vi "BallShear_PackageAnalysis.vi"(4 "Real Coordinates":path=path "C:/Users/Nicole/Documents/GitHub/Ball_Shear/0_BallShear/data/rcoord.csv", 5 "Virtual Coordinates":path=path "C:/Users/Nicole/Documents/GitHub/Ball_Shear/0_BallShear/data/vcoord.csv", 6 "Coord Conversion Script":path=path "C:/Users/Nicole/Documents/GitHub/Ball_Shear/0_BallShear/scripts/coordinate_conversion.py", 7 "Package Analysis Script":path=path "C:/Users/Nicole/Documents/GitHub/Ball_Shear/0_BallShear/scripts/pixel_location.py", 9 "Analyzed Package Path":path=path "C:/Users/Nicole/Documents/GitHub/Ball_Shear/0_BallShear/img/packageAnalyzed.png", 10 "Original Package Path":path=path "C:/Users/Nicole/Documents/GitHub/Ball_Shear/0_BallShear/img/package.png", 11 "Analyze":bool) -> (0 "Displayed Path":path, 1 "IDs":string[](array[string]), 2 "Coordinates":dbl[][](array[numeric]), 3 "Success":bool)   [LabVIEW 2013]
uses:
  <vilib>/Utility/file.llb/Read From Spreadsheet File (DBL).vi
panel:
  out "all rows":dbl[][](array[numeric]) format="%0.3f"
  out "return code 2":i32
  out "standard error 2":string
  out "standard output 2":string
  out "Command 2":string
  out "Command":string
  out "return code":i32
  out "standard error":string
  out "standard output":string
  # "Ball Detection"
  # "Coordinate Conversion"
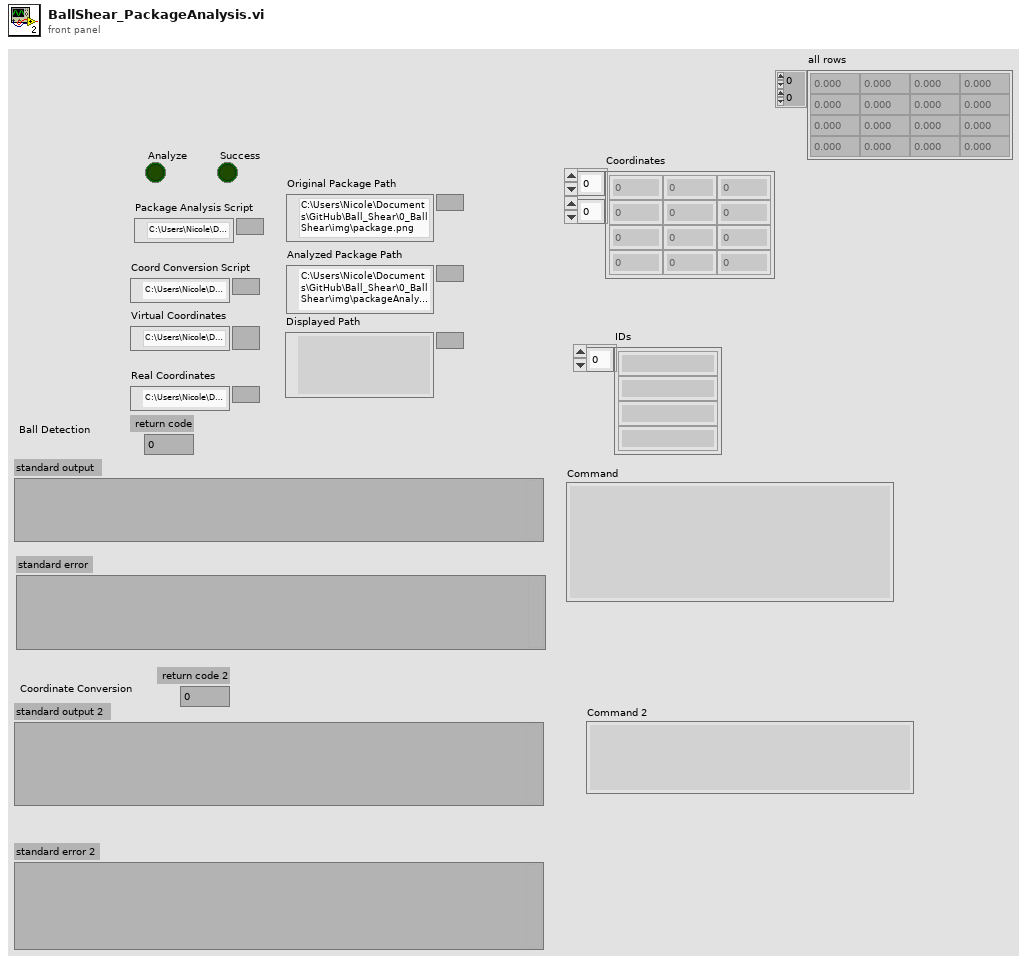
[diagram p1: front panel]
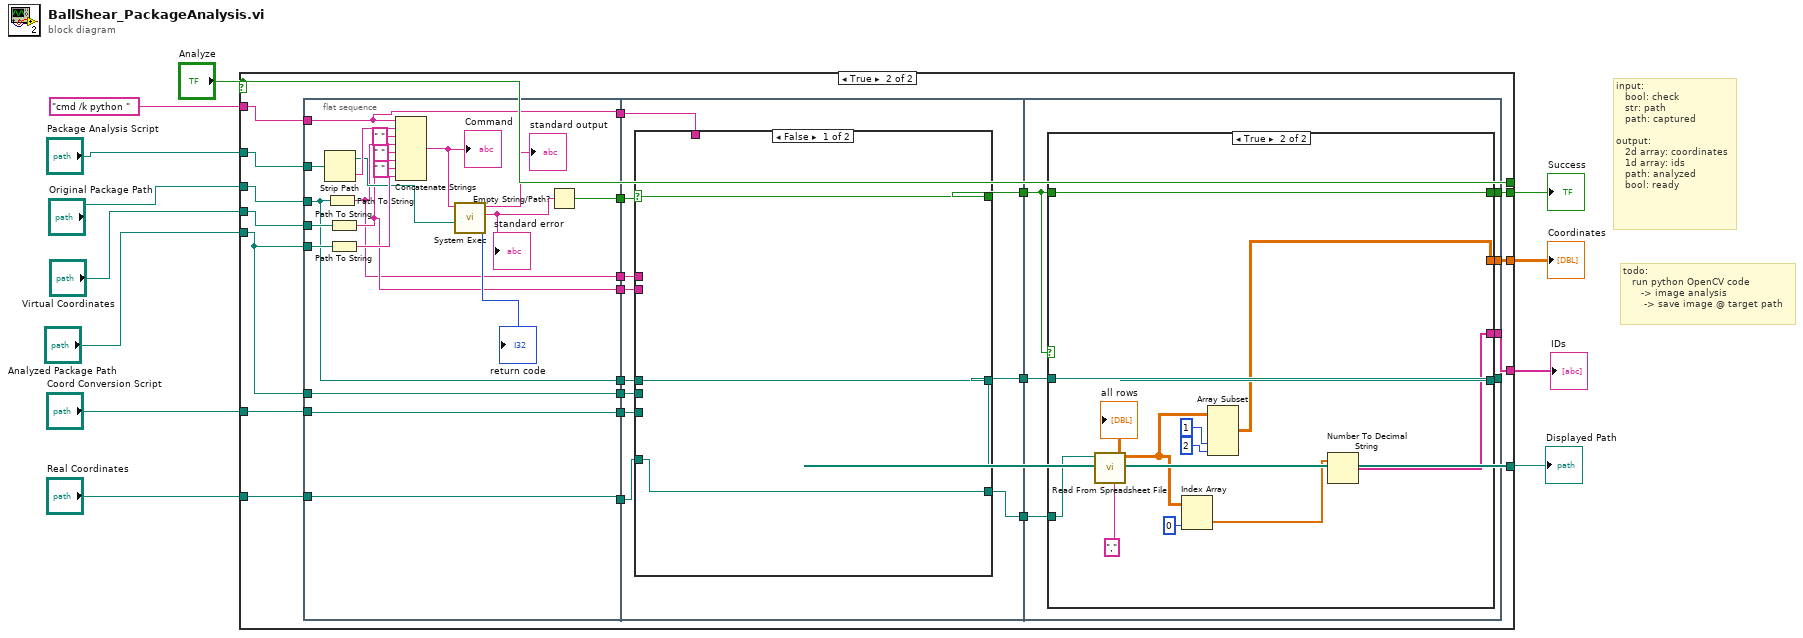
[diagram p0: block diagram]
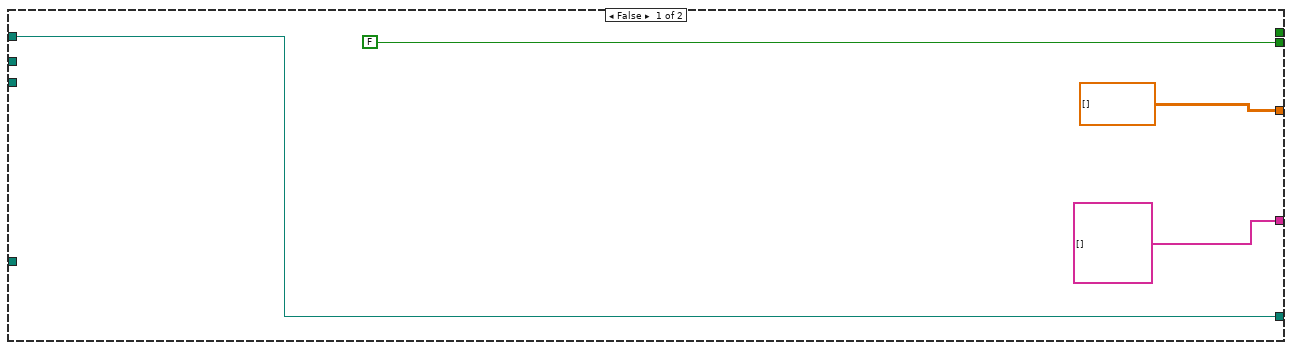
[diagram p2: hidden frame]
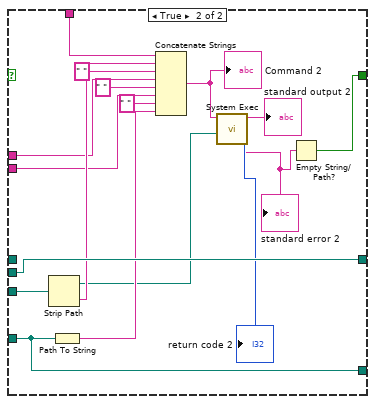
[diagram p3: hidden frame]
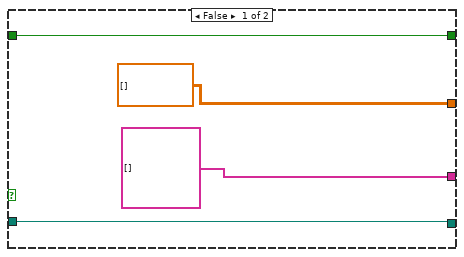
[diagram p4: hidden frame]
diagram:
  # "todo:\n   run python OpenCV code\n      -> image analysis\n       -> save image @ target path"
  # "input:\n   bool: check\n   str: path\n   path: captured\n\noutput:\n   2d array: coordinates\n   1d array: ids\n   path: analyzed\n   bool: ready"
  n1 = case shown="True" "Analyze" {
    tunnel: "Analyze" -> [_ _]
    tunnel: [FALSE ("Power") w32] -> w11
    tunnel: [dbl[][] [] ("Coordinates") w19] -> w10
    tunnel: [string[] [] ("IDs") w18] -> w9
    tunnel: "Original Package Path" -> [w13 w30]
    tunnel: [w13 w27] -> w7
    tunnel: "cmd /k python " -> [_ w38]
    tunnel: "Package Analysis Script" -> [_ w37]
    tunnel: "Virtual Coordinates" -> [_ w36]
    tunnel: "Analyzed Package Path" -> [_ w28]
    tunnel: "Coord Conversion Script" -> [_ w34]
    tunnel: "Real Coordinates" -> [_ w24]
    frame False {
    }
    frame True {
      n2 = flat-sequence {
        tunnel: w38 -> [w42]
        tunnel: w37 -> [w59]
        tunnel: w36 -> [w55]
        tunnel: w28 -> [w54]
        tunnel: [w46] -> w35
        tunnel: w34 -> [w45]
        tunnel: [w45] -> w33
        tunnel: [w44] -> w31
        tunnel: w30 -> [w44]
        tunnel: [w43] -> w29
        tunnel: w28 -> [w43]
        tunnel: [w42] -> w26
        tunnel: [w41] -> w25
        tunnel: w24 -> [w41]
        tunnel: [w40] -> w23
        tunnel: [w39] -> w22
        tunnel: w35 -> [w70]
        tunnel: w33 -> [w69]
        tunnel: w31 -> [w67]
        tunnel: w29 -> [w66]
        tunnel: w26 -> [w64]
        tunnel: w25 -> [w63]
        tunnel: w23 -> [w62]
        tunnel: w22 -> [w61]
        tunnel: [w68] -> w21
        tunnel: [w65] -> w20
        tunnel: [w60] -> w17
        tunnel: [w95] -> w27
        tunnel: [w97] -> w32
        tunnel: w21 -> [w91]
        tunnel: w20 -> [w96]
        tunnel: [w94] -> w19
        tunnel: [w93] -> w18
        tunnel: w17 -> [w92]
        frame #0 {
          n3 = Strip Path(path=w59) -> (stripped path=w50:path, name=w58:string)
          n4 = Path To String(path=w44) -> (string=w39:string)
          n5 = Path To String(path=w55) -> (string=w40:string)
          n6 = Path To String(path=w54) -> (string=w52:string)
          n7 = Concatenate Strings(w42, w58, " " ("string"), w39, " " ("string"), w40, " " ("string"), w52) -> (w51:string)
          "Command" <- w51
          n8 = call <vilib>:"System Exec.vi"("working directory"=w50, "command line"=w51) -> ("return code"=→"return code":i32, "standard error"=w47:string, "standard output"=→"standard output":string)  [unwired: 6 in, 1 out]
          "standard error" <- w47
          n9 = Empty String/Path?(string/path=w47) -> (empty?=w46:bool)
        }
        frame #1 {
          n10 = case shown="False" w70 {
            selector: w70 -> [w73 _]
            tunnel: [w73 w75] -> w68
            tunnel: w69 -> [_ w90]
            tunnel: w67 -> [w72 _]
            tunnel: w66 -> [_ w89]
            tunnel: [w72 w89] -> w65
            tunnel: w64 -> [_ w88]
            tunnel: w63 -> [w71 w74]
            tunnel: w62 -> [_ w83]
            tunnel: w61 -> [_ w85]
            tunnel: [w71 w74] -> w60
            frame False {
            }
            frame True {
              n11 = Strip Path(path=w90) -> (stripped path=w79:path, name=w87:string)
              n12 = Path To String(path=w74) -> (string=w81:string)
              n13 = Concatenate Strings(w88, w87, " " ("string"), w85, " " ("string"), w83, " " ("string"), w81) -> (w80:string)
              "Command 2" <- w80
              n14 = call <vilib>:"System Exec.vi"("working directory"=w79, "command line"=w80) -> ("return code"=→"return code 2":i32, "standard error"=w76:string, "standard output"=→"standard output 2":string)  [unwired: 6 in, 1 out]
              "standard error 2" <- w76
              n15 = Empty String/Path?(string/path=w76) -> (empty?=w75:bool)
            }
          }
        }
        frame #2 {
          n16 = case shown="True" w91 {
            tunnel: [w101 w112] -> w97
            tunnel: w91 -> [w101 w112]
            tunnel: [w100 w111] -> w95
            tunnel: w96 -> [w100 w111]
            tunnel: [dbl[][] [] ("Coordinates") w104] -> w94
            tunnel: [string[] [] ("IDs") w106] -> w93
            tunnel: w92 -> [_ w110]
            frame False {
            }
            frame True {
              n17 = call-poly <vilib>:"Read From Spreadsheet File.vi"("delimiter (\\t)"="," ("delimiter (\\t)"), "file path (dialog if empty)"=w110) -> ("all rows"=w105:dbl[][])  [unwired: 5 in, 4 out]
              "all rows" <- w105
              n18 = Index Array(array=w105, index (col)=0 ("disabled index (col)")) -> (element=w107:dbl[])  [unwired: 1 in]
              n19 = Array Subset(array=w105, index (col)=1 ("index (row)"), length (col)=2 ("length")) -> (w104:dbl[][])  [unwired: 2 in]
              n20 = Number To Decimal String(number=w107) -> (decimal integer string=w106:string[])  [unwired: 1 in]
            }
          }
        }
      }
    }
  }
  "Success" <- w11
  "Coordinates" <- w10
  "IDs" <- w9
  "Displayed Path" <- w7
